vi "CMD Install Graphviz.vi"() -> ()   [LabVIEW 2020]
panel:
  out "standard output":string
  out "standard error":string
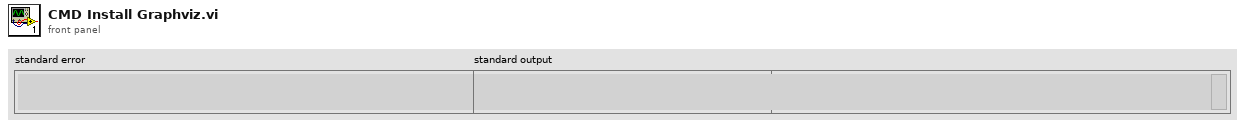
[diagram p1: front panel]
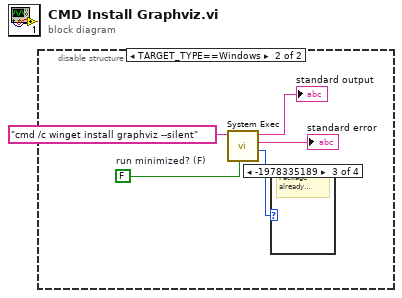
[diagram p0: block diagram]
diagram:
  n1 = disable-structure shown="TARGET_TYPE==Windows" {
    frame condition #0 {
    }
    frame condition #1 (active) {
      w4 = FALSE  # run minimized? (F)
      n2 = call <vilib>:"System Exec.vi"("run minimized? (F)"=w4, "command line"="cmd /c winget install graphviz --silent") -> ("return code"=w3:i32, "standard error"=→"standard error":string, "standard output"=→"standard output":string)  [unwired: 6 in, 1 out]
      n3 = case shown="-1978335189" w3 {
        frame 0 {
        }
        frame Default {
        }
        frame -1978335189 {
          # "Package already installed"
        }
        frame -1978335157 {
          # "No Internet"
        }
      }
    }
  }
